vi "Digital Read Multiple Channels.vi"(8 "error in (no error)":errorcluster, 10 "indices":i32[](array[numeric]), 11 "I-O in":refnum<class "I-O.lvclass">) -> (0 "error out":errorcluster, 2 "Array 2":bool[](array[boolean]), 3 "I-O out":refnum<class "I-O.lvclass">)   [LabVIEW 2021, in "I-O.lvclass"]
uses:
  I-O.lvclass
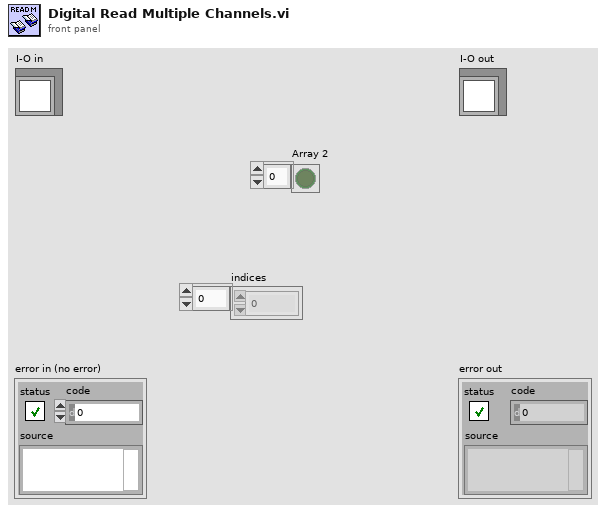
[diagram p1: front panel]
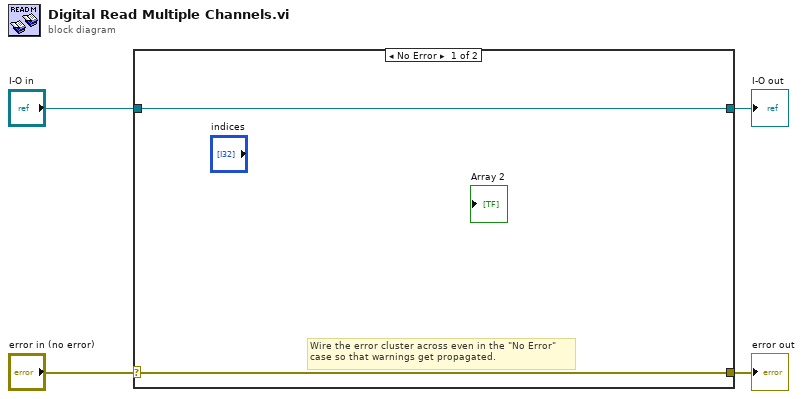
[diagram p0: block diagram]
diagram:
  n1 = case shown="No Error" "error in (no error)" {
    selector: "error in (no error)" -> [w5 w8]
    tunnel: [w5 w8] -> w3
    tunnel: [w6 w7] -> w1
    tunnel: "I-O in" -> [w6 w7]
    frame No Error {
      # "Wire the error cluster across even in the \"No Error\"\ncase so that warnings get propagated."
    }
    frame Error {
    }
  }
  "error out" <- w3
  "I-O out" <- w1
